vi "API_Init Home.vi"(8 "error in (no error)":errorcluster, 11 "Bypass?":bool) -> (0 "error out":errorcluster)   [LabVIEW 2015, in "Tool Module.lvlib"]
doc: "Starts the find home sequence. The tool will move the probe head until it reaches the Reverse limit switch and then back off a short distance. Then it slowly approaches the switch until it just trips. It then resets the encoder to 0 to establish the home position. Once the tool has been homed, the Home bit is set in the Status Byte and the Tool Module reports that the tool is 'Ready'.\n\nThe 'Bypass?' input is used to skip the actual home sequence. If the tool has not been homed since power up, the home bit in the Status byte will still not be set, but the Tool Module will report that the tool is 'Ready'. \n\nOnce the tool has been homed, the homed status bit remains true until power is removed. So, the 'Bypass? input is normally used only after the tool has been homed to get the Tool Module to enter 'Ready' State with out having to re-home the tool."
uses:
  Tool Module.lvlib
  Support/_GoTo Cmd Typedef--enum.ctl
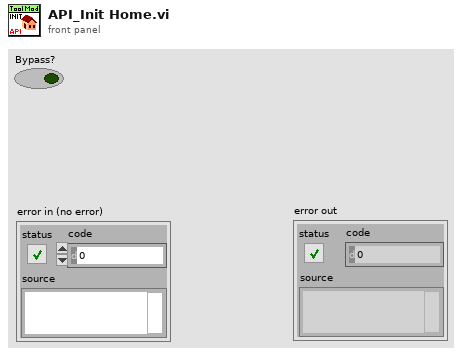
[diagram p1: front panel]
types:
  T1 = typedef "Tool Module.lvlib/_GoTo Cmd Typedef--enum.ctl" = enum16{"MoveA", "MoveR", "Home Position", "Home None", "Cleaning Position"}
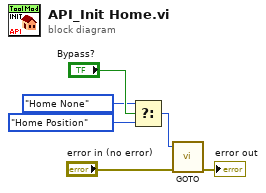
[diagram p0: block diagram]
diagram:
  n1 = Select(t=_GoTo_Cmd_Typedef--enum."Home None" ("_GoTo Cmd typedef"), s="Bypass?", f=_GoTo_Cmd_Typedef--enum."Home Position" ("_GoTo Cmd typedef")) -> (s? t:f=w4:T1)
  n2 = call "GOTO.vi"("error in (no error)"="error in (no error)", "GoTo Cmd"=w4) -> ("error out"=→"error out":errorcluster)  [unwired: 9 in]
